vi "init.vi"(8 "error in":errorcluster, 10 "TBM module configuration in":refnum<class "TBM module configuration.lvclass">, 11 "SystemLin Tag Module runtime in":refnum<class "SystemLink runtime.lvclass">) -> (0 "error out":errorcluster, 1 "data allocations":T1, 2 "execution settings":T4, 3 "SystemLin Tag Module runtime out":refnum<class "SystemLink runtime.lvclass">)   [LabVIEW 2015, in "SystemLink runtime.lvclass"]
doc: "Provides an interface for initializing a module at runtime. While this interface performs no operations, a child should provide an override which may open any necessary references or sessions, allocate necessary memory, and perform any final configuration validataion before providing the full configuration <b>execution data</b> to the calling process."
uses:
  SystemLink runtime.lvclass
  <vilib>/NI/Tag Bus Module Framework/module configuration/TBM module configuration.lvclass
  <vilib>/NI/Tag Bus Module Framework/runtime/execution settings.ctl
  <vilib>/NI/Tag Bus Module Framework/channel/data tables.ctl
  <vilib>/NI/Tag Bus/dictionary/data dictionary.lvclass
  <vilib>/NI/Tag Bus/dictionary table pair.ctl
  <vilib>/NI/Tag Bus/table/data table.ctl
  configuration/SystemLink configuration.lvclass
  configuration/SystemLink configuration.lvclass/SystemLink configuration.ctl
  SystemLink runtime.lvclass/SystemLink runtime.ctl
  configuration/SysLink Mapping.ctl
  configuration/Data Tag Type.ctl
  <vilib>/Skyline/Tag/Wrapper/Wrapper_class/NI Skyline Tag.lvclass
  <vilib>/NI/Tag Bus/tag/tag descriptor.lvclass/tag descriptor.ctl
  <vilib>/NI/Tag Bus Module Framework/channel/TBM channel.lvclass/TBM channel.ctl
  <vilib>/NI/Tag Bus/tag/read tag name.vi
  <vilib>/NI/Tag Bus Module Framework/channel/Read channel classification.vi
  <vilib>/NI/Tag Bus Module Framework/channel/TBM channel.lvclass
  <vilib>/NI/Tag Bus Module Framework/runtime/TBM module execution interface.lvclass
  <vilib>/NI/Tag Bus/tag bus.lvlib
  <vilib>/NI/Tag Bus/table/data table.lvlib
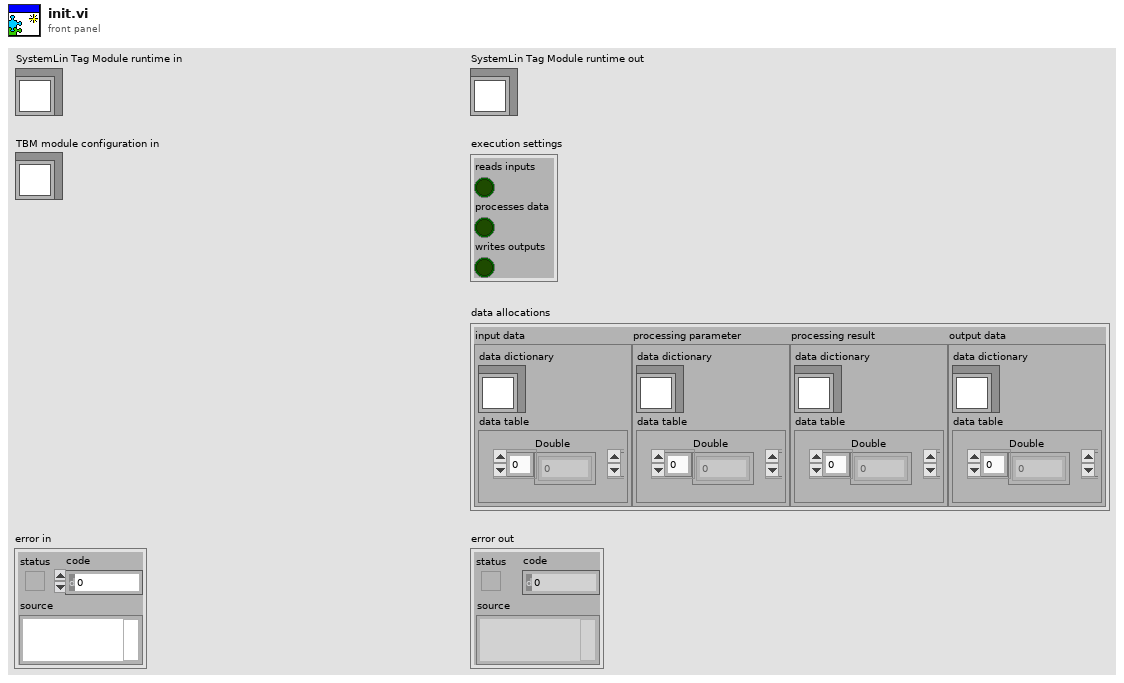
[diagram p1: front panel]
types:
  T1 = typedef "TBM channel.lvclass/data tables.ctl" = cluster{"input data":T2, "processing parameter":T2, "processing result":T2, "output data":T2}
  T2 = typedef "tag bus.lvlib/dictionary table pair.ctl" = cluster{"data dictionary":refnum<class "data dictionary.lvclass">, "data table":T3}
  T3 = typedef "tag bus.lvlib/data table.lvlib/data table.ctl" = cluster{"Double":dbl[], "Single":sgl[], "I64":i64[], "I32":i32[], "I16":i16[], "I8":i8[], "U64":u64[], "U32":u32[], "U16":u16[], "U8":u8[], "Boolean":bool[], "String":string[], "Array of Double":cluster{"DBL Array":dbl[]}[], "Array of Single":cluster{"SGL Array":sgl[]}[], "Array of I64":cluster{"I64 Array":i64[]}[], "Array of I32":cluster{"I32 Array":i32[]}[], "Array of I16":cluster{"I16 Array":i16[]}[], "Array of I8":cluster{"I8 Array":i8[]}[], "Array of U64":cluster{"U64 Array":u64[]}[], "Array of U32":cluster{"U32 Array":u32[]}[], "Array of U16":cluster{"U16 Array":u16[]}[], "Array of U8":cluster{"U8 Array":u8[]}[], "Array of Boolean":cluster{"Boolean Array":bool[]}[], "Array of String":cluster{"String Array":string[]}[]}
  T4 = typedef "TBM module execution interface.lvclass/execution settings.ctl" = cluster{"reads inputs":bool, "processes data":bool, "writes outputs":bool}
  T5 = typedef "SystemLink configuration.lvclass/SysLink Mapping.ctl" = cluster{"Data Type":T6, "Tag Reference":refnum<class "NI Skyline Tag.lvclass">, "Tag Bus Index":i32, "AMQP":bool, "Skylink Index":i32}
  T6 = typedef "SystemLink configuration.lvclass/Data Tag Type.ctl" = enum16{"Double", "Single", "I32", "I16", "I8", "U64", "U32", "U16", "U8", "Boolean", "String", "Timestamp"}
  T7 = typedef "SystemLink configuration.lvclass/Line.ctl" = cluster{"channel":refnum<class "TBM channel.lvclass">, "Data Tag Type":T6}
  T8 = typedef "SystemLink configuration.lvclass/Connection Configuration.ctl" = cluster{"Connection Type":T9, "AMQP":cluster{"Configuration ID":string}, "HTTP":cluster{"Verify Server?":bool, "Server URL":string, "CA Certificate File":string, "User Info":cluster{"Username":string, "Password":string}, "API Key":string}}
  T9 = typedef "SystemLink configuration.lvclass/Connection Type.ctl" = enum16{"AMQP", "HTTP", "API Key (SystemLink Cloud)"}
  T10 = typedef "TBM channel.lvclass/channel classification.ctl" = enum16{"input data", "output data", "processing parameter", "processing result"}
  T11 = typedef "NI Skyline Tag.lvclass/Tag Value Cluster Wrapper.ctl" = cluster{"Configuration":refnum<class "NI Skyline Configuration.lvclass">, "Tag Cluster":T12}
  T12 = typedef "NI Skyline Tag.lvlib/Tag Value Cluster.ctl" = cluster{"Path":string, "Data Type":T13, "Value":string, "Time Stamp":timestamp}
  T13 = typedef "NI Skyline Tag.lvlib/DataType.ctl" = enum32{"Double", "I32", "String", "Boolean", "U64", "Timestamp"}
  T14 = typedef "tag bus.lvlib/tag descriptor.lvclass/Data Type.ctl" = enum16{"Double", "Single", "I64", "I32", "I16", "I8", "U64", "U32", "U16", "U8", "Boolean", "String", "Array of Double", "Array of Single", "Array of I64", "Array of I32", "Array of I16", "Array of I8", "Array of U64", "Array of U32", "Array of U16", "Array of U8", "Array of Boolean", "Array of String"}
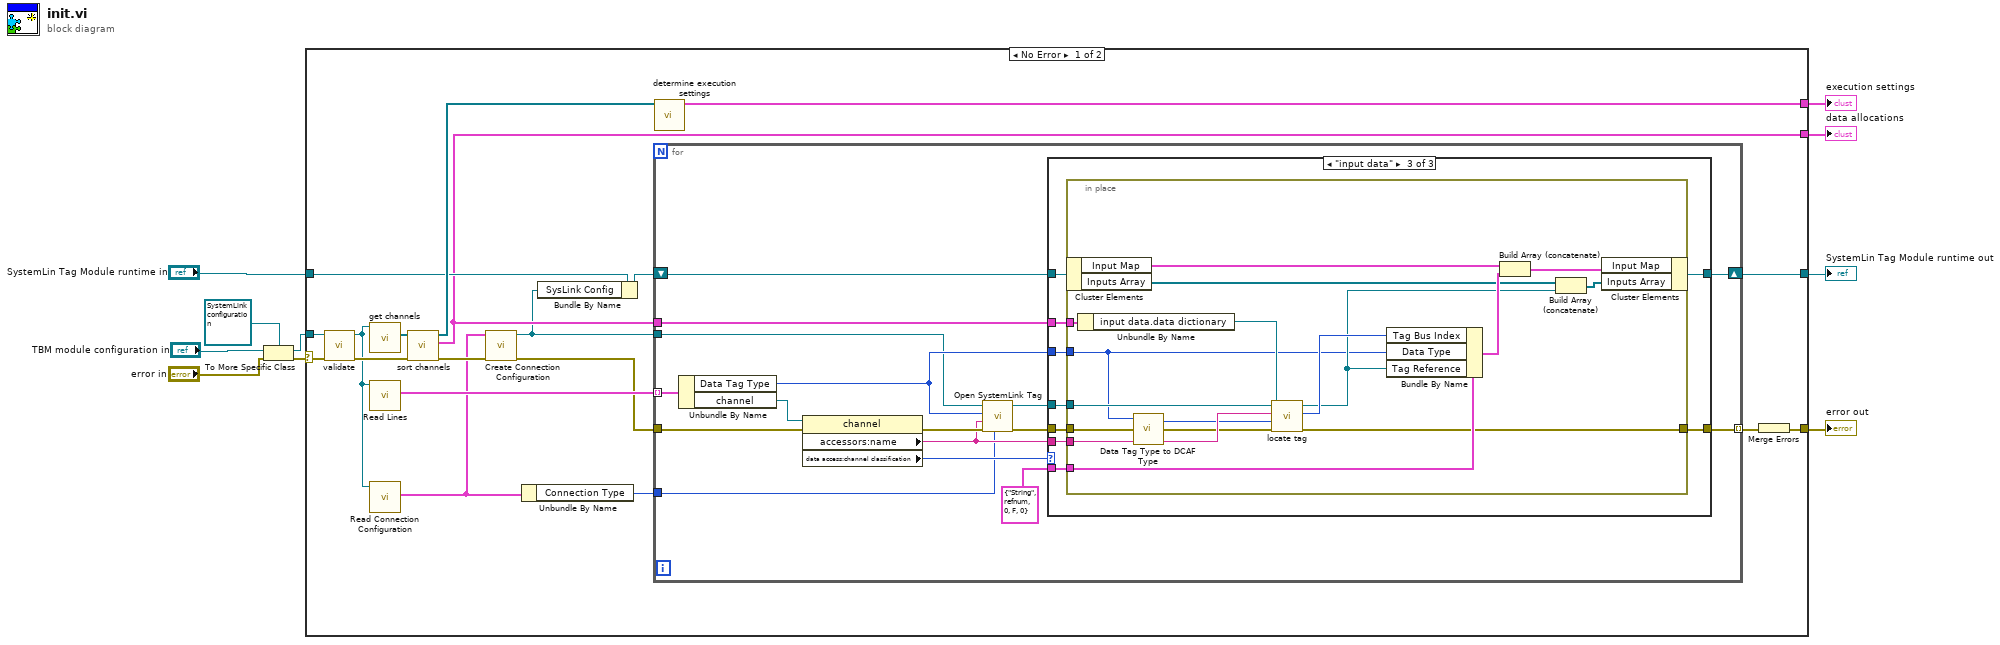
[diagram p0: block diagram]
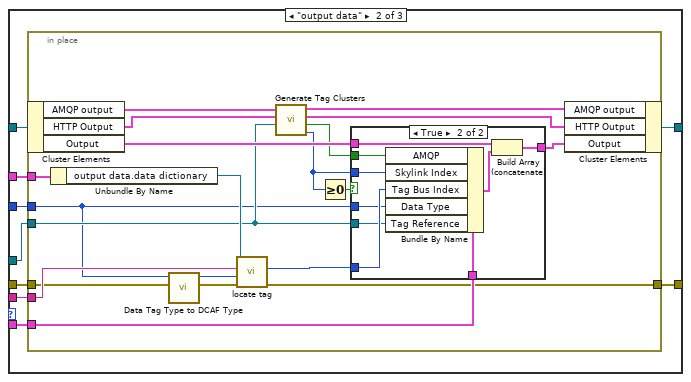
[diagram p3: hidden frame]
diagram:
  n1 = To More Specific Class(target class=refnum<class "SystemLink configuration.lvclass"> refnum ("Synchronous module configuration"), reference="TBM module configuration in", error in="error in") -> (specific class reference=w9:refnum<class "SystemLink configuration.lvclass">, error out=w10:errorcluster)
  n2 = case shown="No Error" w10 {
    selector: w10 -> [w27 w110]
    tunnel: w9 -> [w26 _]
    tunnel: "SystemLin Tag Module runtime in" -> [w23 w111]
    tunnel: [w22 w111] -> w4
    tunnel: [w18 w110] -> w3
    tunnel: [w21 _] -> w1
    tunnel: [w29 _] -> w2
    frame No Error {
      n3 = call-dynamic "validate.vi"("error in"=w27, "SystemLin Tag Module configuration in"=w26) -> ("error out"=w28:errorcluster, "SystemLin Tag Module configuration out"=w15:refnum<class "SystemLink configuration.lvclass">)  [unwired: 8 in]
      n4 = call-dynamic "get channels.vi"("SystemLin Tag Module configuration in"=w15) -> ("channels"=w25:refnum<class "TBM channel.lvclass">[])  [unwired: 9 in, 1 out]
      n5 = call "Read Lines.vi"("SystemLin Tag Module configuration in"=w15) -> ("Lines"=w17:T7[])  [unwired: 8 in, 2 out]
      n6 = call "Read Connection Configuration.vi"("SystemLink configuration in"=w15) -> ("Connection Configuration"=w14:T8)  [unwired: 8 in, 2 out]
      n7 = call <vilib>:"sort channels.vi"("error in"=w28, "channels in"=w25) -> ("error out"=w20:errorcluster, "data allocations"=w21:T1, "channels out"=w24:refnum<class "TBM channel.lvclass">[])  [unwired: 7 in]
      n8 = call "Create Connection Configuration.vi"("error in (no error)"=w20, "Connection Configuration"=w14) -> ("error out"=w16:errorcluster, "SystemLink Configuration"=w11:refnum<class "NI Skyline Configuration.lvclass">)  [unwired: 8 in]
      n9 = Unbundle By Name(w14) -> ("Connection Type"=w13:T9)
      n10 = Bundle By Name(cluster=w23, "SysLink Config"=w11) -> (w12:refnum<class "SystemLink runtime.lvclass">)
      n11 = for {
        shift-right: [w44] -> w22
        shift-left: w12 -> [w45]
        tunnel: w21 -> [w43]
        tunnel: w16 -> [w42]
        tunnel: [w41] -> w19 mode=indexing
        tunnel: w17 -> [w34] mode=indexing
        tunnel: w11 -> [w31]
        tunnel: w13 -> [w30]
        n12 = Unbundle By Name(w34) -> ("Data Tag Type"=w32:T6, "channel"=w33:refnum<class "TBM channel.lvclass">)
        n13 = property class="channel"(reference=w33, error in=w42) -> (error out=w38:errorcluster, "accessors:name"=w36:string, "data access:channel classification"=w35:T10)  [unwired: 1 out]
        n14 = call "Open SystemLink Tag.vi"("Connection Type"=w30, "error in (no error)"=w38, "Path"=w36, "Data Tag Type"=w32, "NI Skyline Configuration in"=w31) -> ("error out"=w37:errorcluster, "NI Skyline Tag out"=w39:refnum<class "NI Skyline Tag.lvclass">)  [unwired: 5 in]
        n15 = case shown="\"input data\"" w35 {
          tunnel: w45 -> [w47 w56 w94]
          tunnel: [w47 w55 w93] -> w44
          tunnel: [w46 w54 w92] -> w41
          tunnel: w37 -> [w46 w53 w91]
          tunnel: T5 {"Data Type"=enum."String", "Tag Reference"=refnum, "Tag Bus Index"=0, "AMQP"=FALSE, "Skylink Index"=0} ("Mapping") -> [_ w52 w90]
          tunnel: w32 -> [_ w51 w89]
          tunnel: w43 -> [_ w50 w88]
          tunnel: w36 -> [_ w49 w87]
          tunnel: w39 -> [_ w48 w86]
          frame Default {
          }
          frame "output data" {
            n16 = in-place {
              in-place-border: w50 -> [w75]
              in-place-border: w49 -> [w70]
              in-place-border: w51 -> [w58]
              in-place-border: w53 -> [w69]
              in-place-border: w52 -> [w68]
              in-place-border: [w67] -> w54
              in-place-border: w48 -> [w66]
              n17 = in-place-cluster #1(w56) -> ("AMQP output"=w65:T11[], "HTTP Output"=w64:T11[], "Output"=w73:T5[])
              n18 = Unbundle By Name(w75) -> ("output data.data dictionary"=w74:refnum<class "data dictionary.lvclass">)
              n19 = call "Data Tag Type to DCAF Type.vi"("Data Tag Type"=w58) -> ("DCAF Data Type"=w57:T14)  [unwired: 10 in]
              n20 = call <vilib>:"locate tag.vi"("error in"=w69, "data type"=w57, "name"=w70, "data dictionary in"=w74) -> ("error out"=w67:errorcluster, "index"=w71:i32)  [unwired: 5 in, 1 out]
              n21 = call "Generate Tag Clusters.vi"("NI Skyline Tag in"=w66, "HTTP Output in"=w64, "AMQP output in"=w65) -> ("Index"=w59:i32, "AMQP"=w61:bool, "HTTP Output out"=w62:T11[], "AMQP output out"=w63:T11[])  [unwired: 5 in]
              n22 = Greater Or Equal To 0?(x=w59) -> (x >= 0?=w60:bool)
              n23 = case shown="True" w60 {
                tunnel: w73 -> [w76 w85]
                tunnel: [w76 w84] -> w72
                tunnel: w71 -> [_ w83]
                tunnel: w68 -> [_ w82]
                tunnel: w58 -> [_ w80]
                tunnel: w66 -> [_ w79]
                tunnel: w59 -> [_ w78]
                tunnel: w61 -> [_ w77]
                frame False {
                }
                frame True {
                  n24 = Bundle By Name(cluster=w82, "AMQP"=w77, "Skylink Index"=w78, "Tag Bus Index"=w83, "Data Type"=w80, "Tag Reference"=w79) -> (w81:T5)
                  n25 = Build Array (concatenate)(w85, w81) -> (w84:T5[])
                }
              }
              n26 = in-place-cluster #1("AMQP output"=w63, "HTTP Output"=w62, "Output"=w72) -> (w55:refnum<class "SystemLink runtime.lvclass">)
            }
          }
          frame "input data" {
            n27 = in-place {
              in-place-border: w88 -> [w109]
              in-place-border: w87 -> [w104]
              in-place-border: w89 -> [w95]
              in-place-border: w91 -> [w103]
              in-place-border: w90 -> [w102]
              in-place-border: [w101] -> w92
              in-place-border: w86 -> [w97]
              n28 = in-place-cluster #2(w94) -> ("Input Map"=w107:T5[], "Inputs Array"=w99:refnum<class "NI Skyline Tag.lvclass">[])
              n29 = Unbundle By Name(w109) -> ("input data.data dictionary"=w108:refnum<class "data dictionary.lvclass">)
              n30 = call "Data Tag Type to DCAF Type.vi"("Data Tag Type"=w95) -> ("DCAF Data Type"=w96:T14)  [unwired: 10 in]
              n31 = call <vilib>:"locate tag.vi"("error in"=w103, "data type"=w96, "name"=w104, "data dictionary in"=w108) -> ("error out"=w101:errorcluster, "index"=w105:i32)  [unwired: 5 in, 1 out]
              n32 = Bundle By Name(cluster=w102, "Tag Bus Index"=w105, "Data Type"=w95, "Tag Reference"=w97) -> (w100:T5)
              n33 = Build Array (concatenate)(w107, w100) -> (w106:T5[])
              n34 = Build Array (concatenate)(w99, w97) -> (w98:refnum<class "NI Skyline Tag.lvclass">[])
              n35 = in-place-cluster #2("Input Map"=w106, "Inputs Array"=w98) -> (w93:refnum<class "SystemLink runtime.lvclass">)
            }
          }
        }
      }
      n36 = call <vilib>:"determine execution settings.vi"("channels"=w24) -> ("execution settings"=w29:T4)  [unwired: 10 in]
      n37 = Merge Errors(w19) -> (w18:errorcluster)
    }
    frame Error {
    }
  }
  "error out" <- w3
  "SystemLin Tag Module runtime out" <- w4
  "execution settings" <- w2
  "data allocations" <- w1
